vi "ER2007 Password Popup Panel.vi"() -> (0 "OK Out":bool, 1 "Super Out":bool)   [LabVIEW 2013]
uses:
  Controls/Global ER2007.vi
panel:
  out "Devel Out":bool
  in  "Password":string
  in  "OK":bool
  # "Utilities Panel access is restricted to privileged users.\n\nPlease enter a password:"
  # "Password"
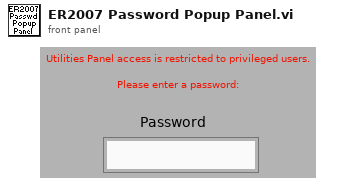
[diagram p1: front panel]
types:
  T1 = enum32{"Invalid", "Standard", "Closed", "Hidden", "Minimized", "Maximized"}
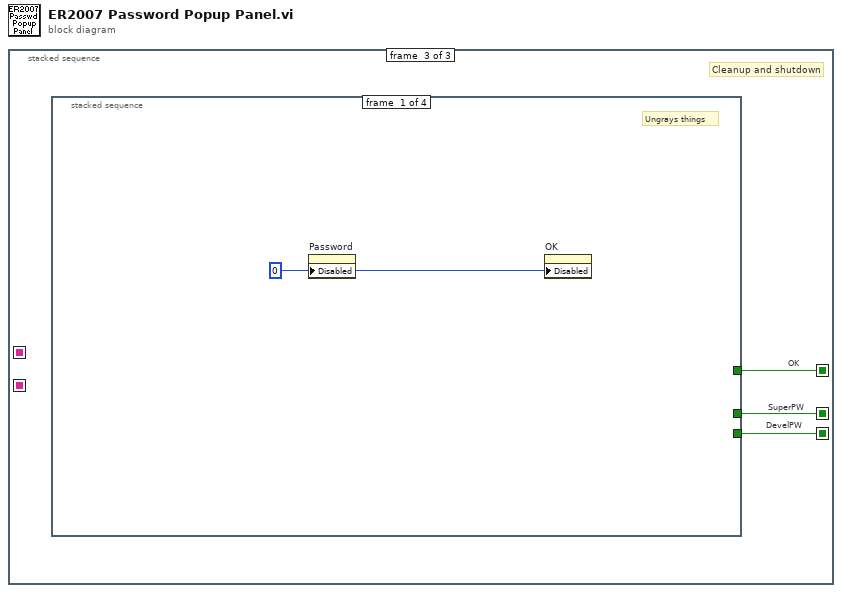
[diagram p0: block diagram]
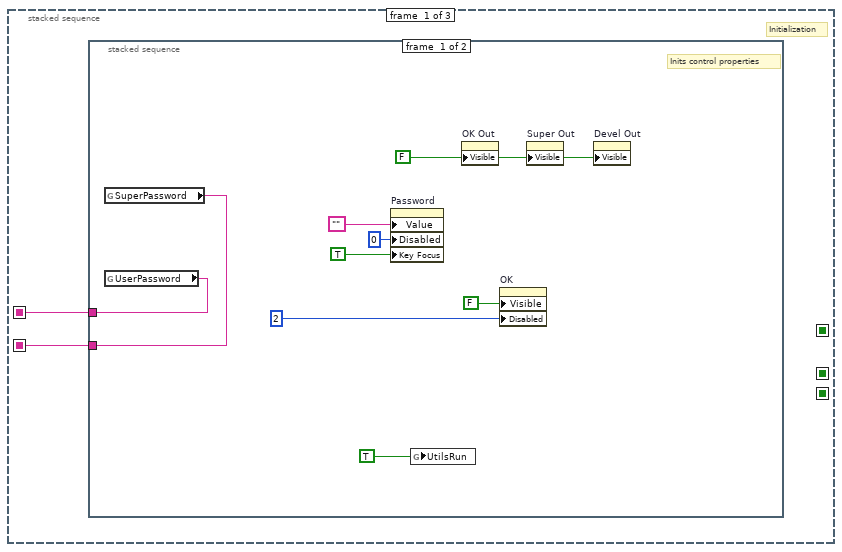
[diagram p2: hidden frame]
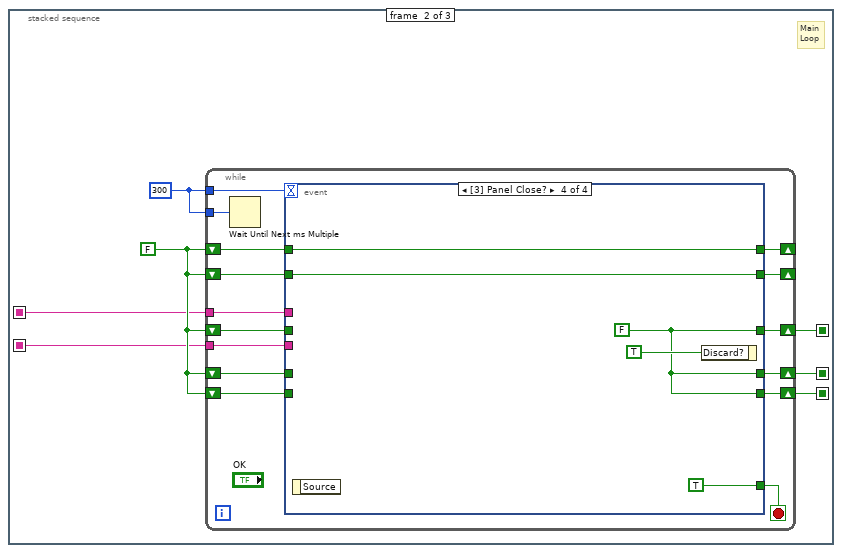
[diagram p4: hidden frame]
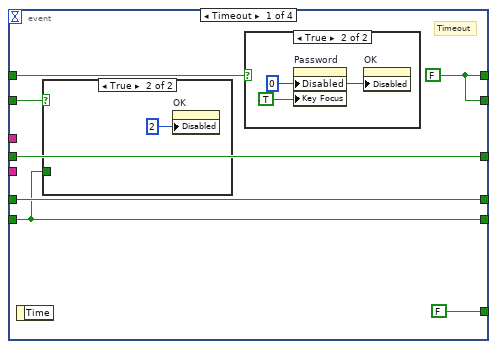
[diagram p5: hidden frame]
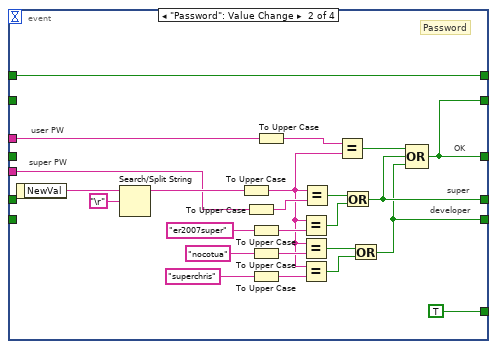
[diagram p8: hidden frame]
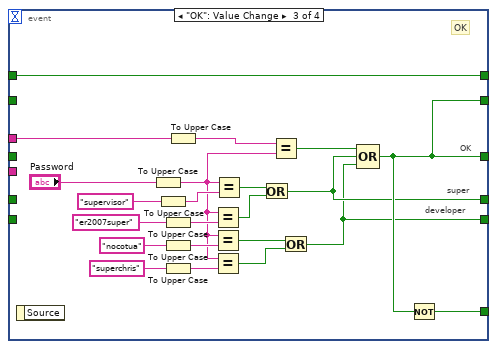
[diagram p9: hidden frame]
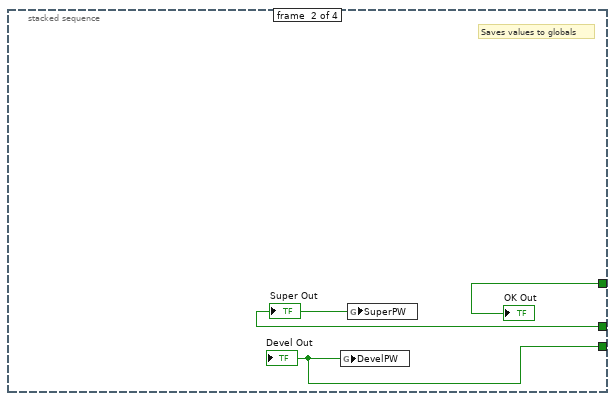
[diagram p10: hidden frame]
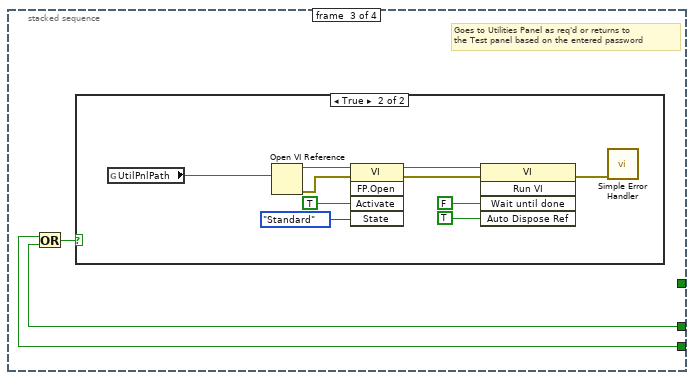
[diagram p11: hidden frame]
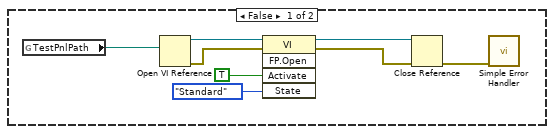
[diagram p12: hidden frame]
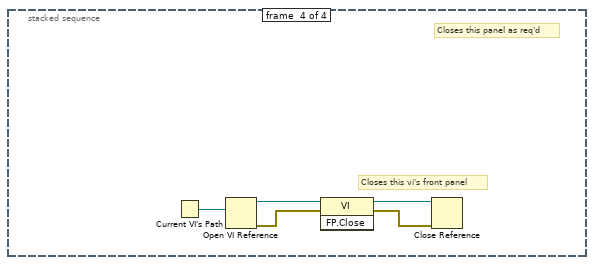
[diagram p13: hidden frame]
diagram:
  n1 = stacked-sequence {
    seq-local: [_ w17 _] -> [_ _ w97]
    seq-local: [_ w16 _] -> [_ _ w96]
    seq-local: [w2 _ _] -> [_ w12 _]
    seq-local: [_ w15 _] -> [_ _ w95]
    seq-local: [w1 _ _] -> [_ w13 _]
    frame #0 {
      # "Initialization"
      n2 = stacked-sequence {
        tunnel: [w5 _] -> w2
        tunnel: [w4 _] -> w1
        frame #0 {
          w9 = FALSE ("Visible")
          # "Inits control properties"
          n3 = global read "Global ER2007.vi" "SuperPassword"() -> (w5:string)
          n4 = global read "Global ER2007.vi" "UserPassword"() -> (w4:string)
          n5 = property on="Password" class="Str"("Value"="", "Disabled"=u8 0, "Key Focus"=TRUE) -> ()  [unwired: 2 in, 2 out]
          n6 = global write "Global ER2007.vi" "UtilsRun"(TRUE ("UtilsRun")) -> ()
          n7 = property on="OK Out" class="Bool (strict)"("Visible"=w9) -> ()  [unwired: 2 in, 2 out]
          n8 = property on="OK" class="Bool"("Visible"=FALSE, "Disabled"=u8 2) -> ()  [unwired: 2 in, 2 out]
          n9 = property on="Super Out" class="Bool (strict)"("Visible"=w9) -> ()  [unwired: 2 in, 2 out]
          n10 = property on="Devel Out" class="Bool (strict)"("Visible"=w9) -> ()  [unwired: 2 in, 2 out]
        }
        frame #1 {
        }
      }
    }
    frame #1 {
      w14 = FALSE
      w18 = u32 300 ("millisecond multiple")
      # "Main\nLoop"
      n11 = while {
        tunnel: w18 -> [w33]
        tunnel: w18 -> [w32]
        shift-right: [w31] -> _
        shift-left: w14 -> [w30]
        shift-right: [w29] -> w17
        shift-left: w14 -> [w23]
        shift-right: [w28] -> w16
        shift-left: w14 -> [w24]
        tunnel: w13 -> [w27]
        shift-right: [w26] -> _
        shift-left: w14 -> [w25]
        shift-right: [w21] -> w15
        shift-left: w14 -> [w20]
        tunnel: w12 -> [w19]
        stop <- w22 stop-if-true
        n12 = Wait Until Next ms Multiple(millisecond multiple=w32) -> ()  [unwired: 1 out]
        n13 = event shown="[3] Panel Close?" {
          selector: _ -> [_ _ _ _]
          dyn-events: _ -> [_ _ _ _]
          timeout: w33 -> [_ _ _ _]
          tunnel: [w38 w58 w82 w94] -> w31
          tunnel: w30 -> [w40 w58 w82 w94]
          tunnel: [w37 w45 w80 w90] -> w29
          tunnel: [w36 w57 w70 w90] -> w28
          tunnel: w27 -> [_ w56 w81 _]
          tunnel: [w38 w45 w80 w93] -> w26
          tunnel: w25 -> [w39 _ _ w93]
          tunnel: w24 -> [w36 _ _ _]
          tunnel: w23 -> [w37 _ _ _]
          tunnel: [FALSE TRUE w79 TRUE] -> w22
          tunnel: [w34 w47 w69 w90] -> w21
          tunnel: w20 -> [w34 _ _ _]
          tunnel: w19 -> [_ w46 _ _]
          event Timeout {
            w38 = FALSE
            # "Timeout"
            n14 = event-data() -> ()  [unwired: 1 in, 1 out]
            n15 = case shown="True" w39 {
              tunnel: w34 -> [_ _]
              frame False {
              }
              frame True {
                n16 = property on="OK" class="Bool"("Disabled"=u8 2) -> ()  [unwired: 2 in, 2 out]
              }
            }
            n17 = case shown="True" w40 {
              frame False {
              }
              frame True {
                w43 = u8 0 ("Disabled")
                n18 = property on="Password" class="Str"("Disabled"=w43, "Key Focus"=TRUE) -> ()  [unwired: 2 in, 2 out]
                n19 = property on="OK" class="Bool"("Disabled"=w43) -> ()  [unwired: 2 in, 2 out]
              }
            }
          }
          event "Password": Value Change {
            # "super PW"
            # "user PW"
            # "developer"
            # "OK"
            # "super"
            # "Password"
            n20 = event-data() -> ("NewVal"=w55:string)  [unwired: 1 in]
            n21 = Search/Split String(string=w55, search string/char (-)="\r") -> (substring before match=w54:string)  [unwired: 1 in, 2 out]
            n22 = To Upper Case(1:w54) -> (0:w59:string)
            n23 = To Upper Case(1:w46) -> (0:w65:string)
            n24 = To Upper Case(1:"er2007super") -> (0:w64:string)
            n25 = To Upper Case(1:"nocotua") -> (0:w61:string)
            n26 = To Upper Case(1:"superchris") -> (0:w60:string)
            n27 = To Upper Case(1:w56) -> (0:w66:string)
            n28 = Equal?(x=w59, y=w64) -> (x = y?=w62:bool)
            n29 = Equal?(x=w59, y=w61) -> (x = y?=w49:bool)
            n30 = Equal?(x=w59, y=w60) -> (x = y?=w48:bool)
            n31 = Equal?(x=w59, y=w65) -> (x = y?=w63:bool)
            n32 = Equal?(x=w66, y=w59) -> (x = y?=w67:bool)
            n33 = Or(x=w63, y=w62) -> (x .or. y?=w57:bool)
            n34 = Or(x=w49, y=w48) -> (x .or. y?=w47:bool)
            n35 = Compound Arithmetic op=OR(w67, w57, w47) -> (w45:bool)
          }
          event "OK": Value Change {
            # "developer"
            # "OK"
            # "super"
            # "OK"
            n36 = event-data() -> ()  [unwired: 1 in, 1 out]
            n37 = To Upper Case(1:"Password") -> (0:w83:string)
            n38 = To Upper Case(1:"supervisor") -> (0:w87:string)
            n39 = To Upper Case(1:"er2007super") -> (0:w86:string)
            n40 = To Upper Case(1:"nocotua") -> (0:w85:string)
            n41 = To Upper Case(1:"superchris") -> (0:w84:string)
            n42 = To Upper Case(1:w81) -> (0:w88:string)
            n43 = Equal?(x=w83, y=w86) -> (x = y?=w71:bool)
            n44 = Equal?(x=w83, y=w85) -> (x = y?=w74:bool)
            n45 = Equal?(x=w83, y=w84) -> (x = y?=w73:bool)
            n46 = Equal?(x=w83, y=w87) -> (x = y?=w72:bool)
            n47 = Or(x=w72, y=w71) -> (x .or. y?=w70:bool)
            n48 = Equal?(x=w88, y=w83) -> (x = y?=w89:bool)
            n49 = Or(x=w74, y=w73) -> (x .or. y?=w69:bool)
            n50 = Compound Arithmetic op=OR(w89, w70, w69) -> (w80:bool)
            n51 = Not(x=w80) -> (.not. x?=w79:bool)
          }
          event Panel Close? {
            w90 = FALSE
            n52 = event-data() -> ()  [unwired: 1 in, 1 out]
            n53 = event-data("Discard?"=TRUE) -> ()  [unwired: 1 in, 1 out]
          }
        }
      }
    }
    frame #2 {
      # "DevelPW"
      # "SuperPW"
      # "OK"
      # "Cleanup and shutdown"
      n54 = stacked-sequence {
        tunnel: w97 -> [_ w101 _ _]
        tunnel: w96 -> [_ w100 w103 _]
        tunnel: w95 -> [_ w99 w102 _]
        frame #0 {
          w98 = u8 0 ("Disabled")
          # "Ungrays things"
          n55 = property on="Password" class="Str"("Disabled"=w98) -> ()  [unwired: 2 in, 2 out]
          n56 = property on="OK" class="Bool"("Disabled"=w98) -> ()  [unwired: 2 in, 2 out]
        }
        frame #1 {
          # "Saves values to globals"
          n57 = global write "Global ER2007.vi" "DevelPW"(w99) -> ()
          n58 = global write "Global ER2007.vi" "SuperPW"(w100) -> ()
          "OK Out" <- w101
          "Super Out" <- w100
          "Devel Out" <- w99
        }
        frame #2 {
          # "Goes to Utilities Panel as req'd or returns to\nthe Test panel based on the entered password"
          n59 = Or(x=w102, y=w103) -> (x .or. y?=w104:bool)
          n60 = case shown="True" w104 {
            frame False {
              n61 = global read "Global ER2007.vi" "TestPnlPath"() -> (w105:path)
              n62 = Open VI Reference(vi path=w105) -> (vi reference=w110:refnum<vi>, error out=w109:errorcluster)  [unwired: 5 in]
              n63 = invoke class="VI" method="FP.Open"(reference=w110, error in=w109, "Activate"=TRUE, "State"=T1."Standard") -> (reference out=w108:refnum<vi>, error out=w107:errorcluster)  [unwired: 1 in, 3 out]
              n64 = Close Reference(reference=w108, error in (no error)=w107) -> (error out=w106:errorcluster)
              n65 = call <vilib>:"Simple Error Handler.vi"("error in (no error)"=w106) -> ()  [unwired: 4 in, 5 out]
            }
            frame True {
              n66 = global read "Global ER2007.vi" "UtilPnlPath"() -> (w113:path)
              n67 = Open VI Reference(vi path=w113) -> (vi reference=w118:refnum<vi>, error out=w116:errorcluster)  [unwired: 5 in]
              n68 = invoke class="VI" method="FP.Open"(reference=w118, error in=w116, "Activate"=TRUE, "State"=T1."Standard") -> (reference out=w119:refnum<vi>, error out=w117:errorcluster)  [unwired: 1 in, 3 out]
              n69 = invoke class="VI" method="Run VI"(reference=w119, error in=w117, "Wait until done"=FALSE, "Auto Dispose Ref"=TRUE) -> (error out=w122:errorcluster)  [unwired: 1 in, 4 out]
              n70 = call <vilib>:"Simple Error Handler.vi"("error in (no error)"=w122) -> ()  [unwired: 4 in, 5 out]
            }
          }
        }
        frame #3 {
          # "Closes this vi's front panel"
          # "Closes this panel as req'd"
          n71 = Current VI's Path() -> (path=w127:path)
          n72 = Open VI Reference(vi path=w127) -> (vi reference=w126:refnum<vi>, error out=w125:errorcluster)  [unwired: 5 in]
          n73 = invoke class="VI" method="FP.Close"(reference=w126, error in=w125) -> (reference out=w124:refnum<vi>, error out=w123:errorcluster)  [unwired: 1 in, 1 out]
          n74 = Close Reference(reference=w124, error in (no error)=w123) -> ()  [unwired: 1 out]
        }
      }
    }
  }
